vi "External Trigger.vi"(4 "front panel trigger out":bool) -> (1 "front panel trigger in":bool)   [LabVIEW 2018, in "GettingStarted_5774_FPGA.lvlib"]
doc: "Front panel TRIG IN and TRIG OUT\n\nConnects the input value to TRIG OUT with a pulse expander to ensure that the signal is visible long enough to be detected by a reasonable target device.\n\nInputs the TRIG IN and adds edge-sensitivity to it to ensure only one trigger is received per external edge."
uses:
  GettingStarted_5774_FPGA.lvlib
  <vilib>/rvi/eio/common/nirviEmuTemplateMethod_errors.vi
  <vilib>/eio/EIONode/EIONode.xnode
  <instrlib>/_niInstr/Basic Elements/v1/FPGA/niInstr Basic Elements v1 FPGA.lvlib
  <instrlib>/FlexRIO/API/FPGA/v1/FlexRIO API FPGA v1.lvlib
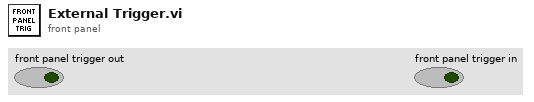
[diagram p1: front panel]
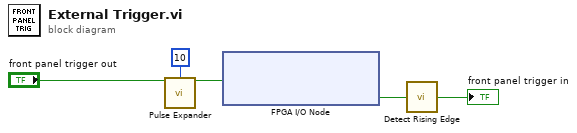
[diagram p0: block diagram]
diagram:
  n1 = call <instrlib>:"Pulse Expander.vi"("input pulse"="front panel trigger out", "min pulse length"=10) -> ("expanded pulse"=w2:bool)  [unwired: 13 in]
  n2 = xnode "FPGA I/O Node"("IO Socket\\TriggerOut"=w2) -> ("IO Socket\\TriggerIn"=w5:bool)  [unwired: 2 in, 2 out]
  n3 = call <instrlib>:"Detect Rising Edge.vi"("signal"=w5) -> ("edge detected"=→"front panel trigger in":bool)  [unwired: 14 in]
